vi "Calculations.system.vi"(8 "Îperator":string, 10 "Number Y":string, 11 "Number X":string) -> (2 "Resalt":string)   [LabVIEW 2020]
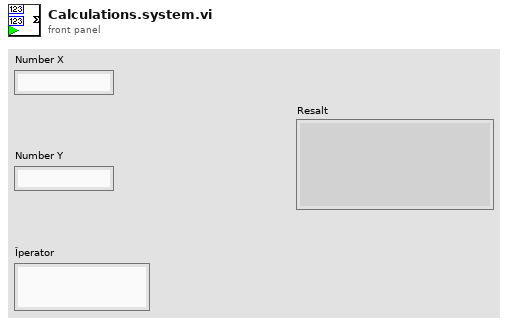
[diagram p1: front panel]
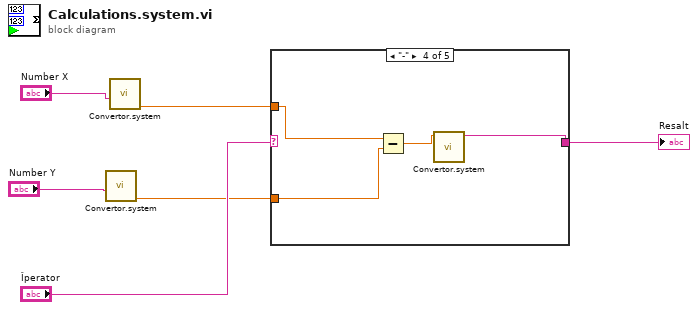
[diagram p0: block diagram]
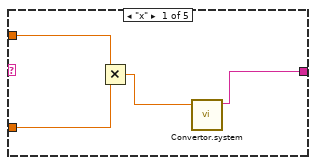
[diagram p2: hidden frame]
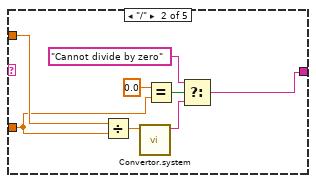
[diagram p3: hidden frame]
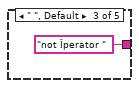
[diagram p4: hidden frame]
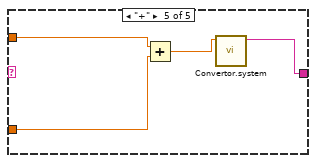
[diagram p5: hidden frame]
diagram:
  n1 = call "Convertor.system.vi"("String"="Number Y") -> ("String to DBL"=w2:dbl)  [unwired: 7 in, 1 out]
  n2 = call "Convertor.system.vi"("String"="Number X") -> ("String to DBL"=w3:dbl)  [unwired: 7 in, 1 out]
  n3 = case shown="\"-\"" "Îperator" {
    tunnel: w3 -> [w10 w18 _ w23 w27]
    tunnel: w2 -> [w9 w15 _ w22 w26]
    tunnel: [w7 w13 "not Îperator " ("f") w20 w24] -> w1
    frame "x" {
      n4 = Multiply(x=w10, y=w9) -> (x*y=w8:dbl)
      n5 = call "Convertor.system.vi"("DBL"=w8) -> ("DBL to string"=w7:string)  [unwired: 7 in, 1 out]
    }
    frame "/" {
      n6 = Divide(x=w18, y=w15) -> (x/y=w14:dbl)
      n7 = call "Convertor.system.vi"("DBL"=w14) -> ("DBL to string"=w11:string)  [unwired: 7 in, 1 out]
      n8 = Equal?(x=0.0, y=w15) -> (x = y?=w16:bool)
      n9 = Select(t="Cannot divide by zero" ("f"), s=w16, f=w11) -> (s? t:f=w13:string)
    }
    frame " ", Default {
    }
    frame "-" {
      n10 = Subtract(x=w23, y=w22) -> (x-y=w21:dbl)
      n11 = call "Convertor.system.vi"("DBL"=w21) -> ("DBL to string"=w20:string)  [unwired: 7 in, 1 out]
    }
    frame "+" {
      n12 = Add(x=w27, y=w26) -> (x+y=w25:dbl)
      n13 = call "Convertor.system.vi"("DBL"=w25) -> ("DBL to string"=w24:string)  [unwired: 7 in, 1 out]
    }
  }
  "Resalt" <- w1
